vi "ModuleCode.vi"(11 "LoggingWrapper in":refnum<class "LoggingWrapper.lvclass">) -> (2 "ModuleCode":string, 3 "LoggingWrapper out":refnum<class "LoggingWrapper.lvclass">)   [LabVIEW 2022 SP3, in "Logger.lvlib" / "LoggingWrapper.lvclass"]
uses:
  LoggingWrapper.lvclass
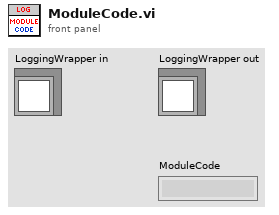
[diagram p1: front panel]
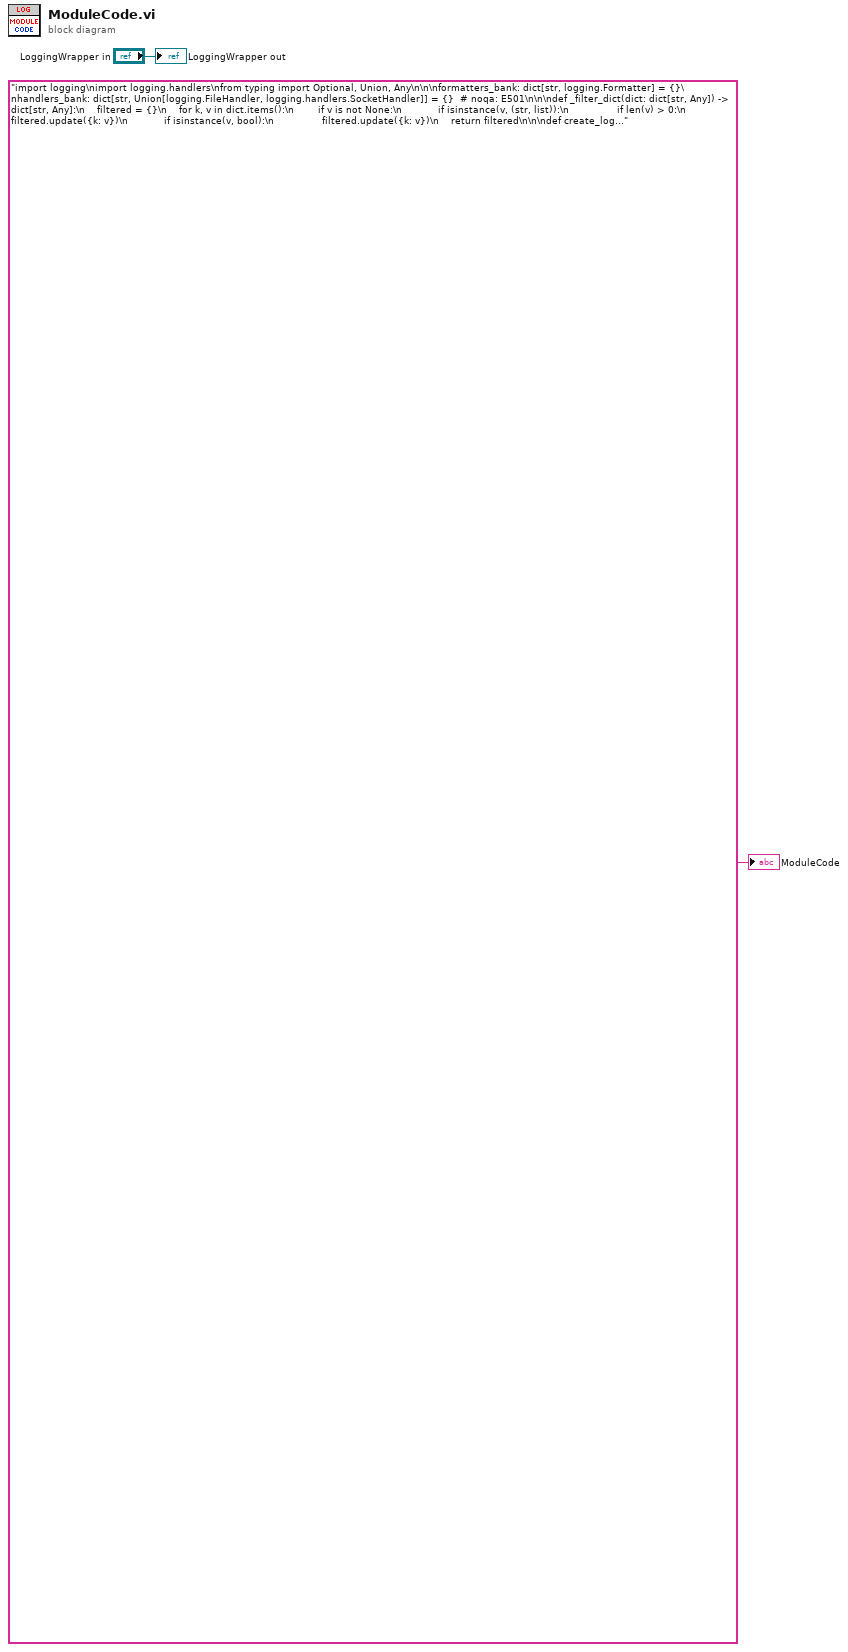
[diagram p0: block diagram]
diagram:
  "LoggingWrapper out" <- "LoggingWrapper in"
  "ModuleCode" <- "import logging\nimport logging.handlers\nfrom typing import Optional, Union, Any\n\n\nformatters_bank: dict[str, logging.Formatter] = {}\nhandlers_bank: dict[str, Union[logging.FileHandler, logging.handlers.SocketHandler]] = {}  # noqa: E501\n\n\ndef _filter_dict(dict: dict[str, Any]) -> dict[str, Any]:\n    filtered = {}\n    for k, v in dict.items():\n        if v is not None:\n            if isinstance(v, (str, list)):\n                if len(v) > 0:\n                    filtered.update({k: v})\n            if isinstance(v, bool):\n                filtered.update({k: v})\n    return filtered\n\n\ndef create_logger(logger_name: str):\n    logging.getLogger(logger_name)\n\n\ndef set_logger_level(logger_name: str, level: str):\n    logging.getLogger(logger_name).setLevel(level)\n\n\ndef create_file_handler(\n        handler_name: str,\n        file_path: str,\n        mode: str = 'a',\n        encoding: Optional[str] = None,\n        delay: bool = False,\n        errors: Optional[str] = None\n        ):\n    kwargs = _filter_dict(locals())\n    name = kwargs.pop('handler_name')\n    filename = kwargs.pop('file_path')\n    global handlers_bank\n    handler = logging.FileHandler(filename=filename, **kwargs)\n    handlers_bank.update({name: handler})\n\n\ndef create_socket_handler(handler_name: str, host: str, port: int):\n    global handlers_bank\n    handler = logging.handlers.SocketHandler(host=host, port=port)\n    handlers_bank.update({handler_name: handler})\n\n\ndef set_handler_level(handler_name: str, level: str):\n    global handlers_bank\n    handlers_bank.get(handler_name).setLevel(level=level)\n\n\ndef add_handler(logger_name: str, handler_name: str):\n    global handlers_bank\n    handler = handlers_bank.get(handler_name)\n    logging.getLogger(logger_name).addHandler(handler)\n\n\ndef create_formatter(\n        formatter_name: str,\n        format: str,\n        date_format: Optional[str],\n        style: Optional[str],\n        validate: bool = True\n        ):\n    kwargs = _filter_dict(locals())\n    name = kwargs.pop('formatter_name')\n    fmt = kwargs.pop('format')\n    datefmt = kwargs.pop('date_format', None)\n    global formatters_bank\n    formatter = logging.Formatter(fmt=fmt, datefmt=datefmt, **kwargs)\n    formatters_bank.update({name: formatter})\n\n\ndef set_formatter(handler_name: str, formatter_name: str):\n    global handlers_bank, formatters_bank\n    handler = handlers_bank.get(handler_name)\n    formatter = formatters_bank.get(formatter_name)\n    handler.setFormatter(formatter)\n\n\ndef info(logger_name: str, message: str):\n    logging.getLogger(logger_name).info(message)\n\n\ndef debug(logger_name: str, message: str):\n    logging.getLogger(logger_name).debug(message)\n\n\ndef warning(logger_name: str, message: str):\n    logging.getLogger(logger_name).warning(message)\n\n\ndef error(logger_name: str, message: str):\n    logging.getLogger(logger_name).error(message)\n\n\ndef critical(logger_name: str, message: str):\n    logging.getLogger(logger_name).critical(message)\n" ("PythonCode")
